vi "Controller Acquisition and Actuation Loop.vi"(4 "Iteration Duration":i64, 5 "Missed iteration?":bool, 6 "Initial Corrector Kick Vector":dbl[](array[numeric]), 7 "Sync Objects":T3, 8 "error in (no error)":errorcluster, 9 "PS Variables":T1, 10 "BPM Variables":T2, 11 "FOFB Configuration":T7={"FOFB Parameters"={"Network"={"FOFB Controller IP"="", "LNLS Control Network IP"="", "LNLS Control Network Power Supplies TCP Port"=0, "LNLS Control Network FOFB Configuration TCP Port"=0, "Data Server TCP Port"=0, "Monitoring Data TCP Port"=0, "Configuration GUI TCP Port"=0, "TCP Listening Timeout"=0}, "Fast Acquisition"={"Acquisition Period"=0, "Data Buffer Size"=0, "Monitoring Period"=0}, "Response Matrix Measurement"={"Step Amplitude"=0.0, "Time Between Steps"=0, "Step Duration"=0, "Number of Averages"=0}, "Correction Algorithm"={"Correction Period"=0, "Reference Orbit Path"=path "", "Response Matrix Path"=path "", "Correction Matrix Path"=path "", "Horizontal Correction Factor"=0.0, "Vertical Correction Factor"=0.0, "Beam Current FOFB Threshold"=0.0, "Decouple H-V"=FALSE, "Use Additional BPM LPF"=FALSE, "BPM LPF Cutoff"=0.0}, "Acquisition Network"=[], "Actuation Network"=[]}, "Number of Acquisition Chassis"=0, "Number of Actuation Chassis"=0, "Number of BPM Readings"=0, "BPM Reading Names"=[], "Selected BPM Readings"=[0, 1, 2, 3, 4, 5, 6, 7, 8, 9, 10, 11, 12, 13, 14, 15, 16, 17, 18, 19, 20, 21, 22, 23, 24, 25, 26, 27, 28, 29, 30, 31, 32, 33, 34, 35, 36, 37, 38, 39, 40, 41, 42, 43, 44, 45, 46, 47, 48, 49], "Number of Correctors"=0, "Corrector Names"=[], "Selected Correctors"=[0, 1, 2, 3, 4, 5, 6, 7, 8, 9, 10, 11, 12, 13, 14, 15, 16, 17, 18, 19, 20, 21, 22, 23, 24, 25, 26, 27, 28, 29, 30, 31, 32, 33, 34, 35, 36, 37, 38, 39, 40, 41, 42, 43, 44, 45, 46, 47, 48, 49], "Reference Orbit"=[], "Response Matrix"=[], "Correction Matrix"=[], "Acquisition Chassis Names"=[], "Actuation Chassis Names"=[], "Acquisition Variables"=[], "Actuation Variables"=[], "PS Matrix Mapping"=[], "Inverse PS Matrix Mapping"=[], "Response Matrix Beam Energy (MeV)"=0.0, "PID Parameters"=[], "BPM Planes"=[], "Corrector Planes"=[], "RMM Step Factor"=[]}) -> (0 "error out":errorcluster)   [LabVIEW 2011, in "Controller VIs.lvlib"]
doc: "Continuously performs acquisition of all input variables (BPM readings, Power Supply readings, etc.) and forwards data to the <b>Decimated Acquisition Loop</b>. Depending on the <b>Actuation State</b> (global variable), performs actuations coming from one of the following sources (global variables):\n\n<b>Actuation State</b> = Only Reading\n (no actuation)\n\n<b>Actuation State</b> = Manual\n PS_Manual_Setpoints\n\n<b>Actuation State</b> = FOFB, Initializing FOFB, Stopping FOFB\n PS_FOFB_Setpoints\n\n<b>Actuation State</b> = Response Matrix Measurement\n PS_RMM_Setpoints"
uses:
  Controller VIs.lvlib
  Types Definitions/Type FOFB Configuration.ctl
  Types Definitions/Type FOFB Parameters.ctl
  Types Definitions/Type Network Configuration.ctl
  Types Definitions/Type FA Configuration.ctl
  Types Definitions/Type Response Matrix Measurement Configuration.ctl
  Types Definitions/Type Correction Algorithm Configuration.ctl
  Types Definitions/Type Acquisition Network Configuration.ctl
  Types Definitions/Type Actuation Network Configuration.ctl
  Types Definitions/Type PID Parameters.ctl
  Types Definitions/Type Synchronization Objects.ctl
  Types Definitions/Type Blocking Synchronization Objects.ctl
  Types Definitions/Type FA Request Parameters.ctl
  Types Definitions/Type BPM and PS select cluster.ctl
  Types Definitions/Type FA File Parameters.ctl
  Types Definitions/Type Monitoring Data.ctl
  Types Definitions/Type Diagnostics Data.ctl
  Types Definitions/Type CPU Loads Array.ctl
  Types Definitions/Type CPU Loads.ctl
  Types Definitions/Type Non-blocking Synchronization Objects.ctl
  Types Definitions/Type FOFB Variables.ctl
  Types Definitions/Type Actuation State.ctl
  Types Definitions/Type BPM Variables.ctl
  Types Definitions/Type PS Variables.ctl
  <vilib>/Analysis/3filter.llb/Filter Passband Type.ctl
  Type Definitions.lvlib
  <vilib>/Analysis/NI_AALBase.lvlib
  <vilib>/ptbypt/NI_PtbyPt.lvlib
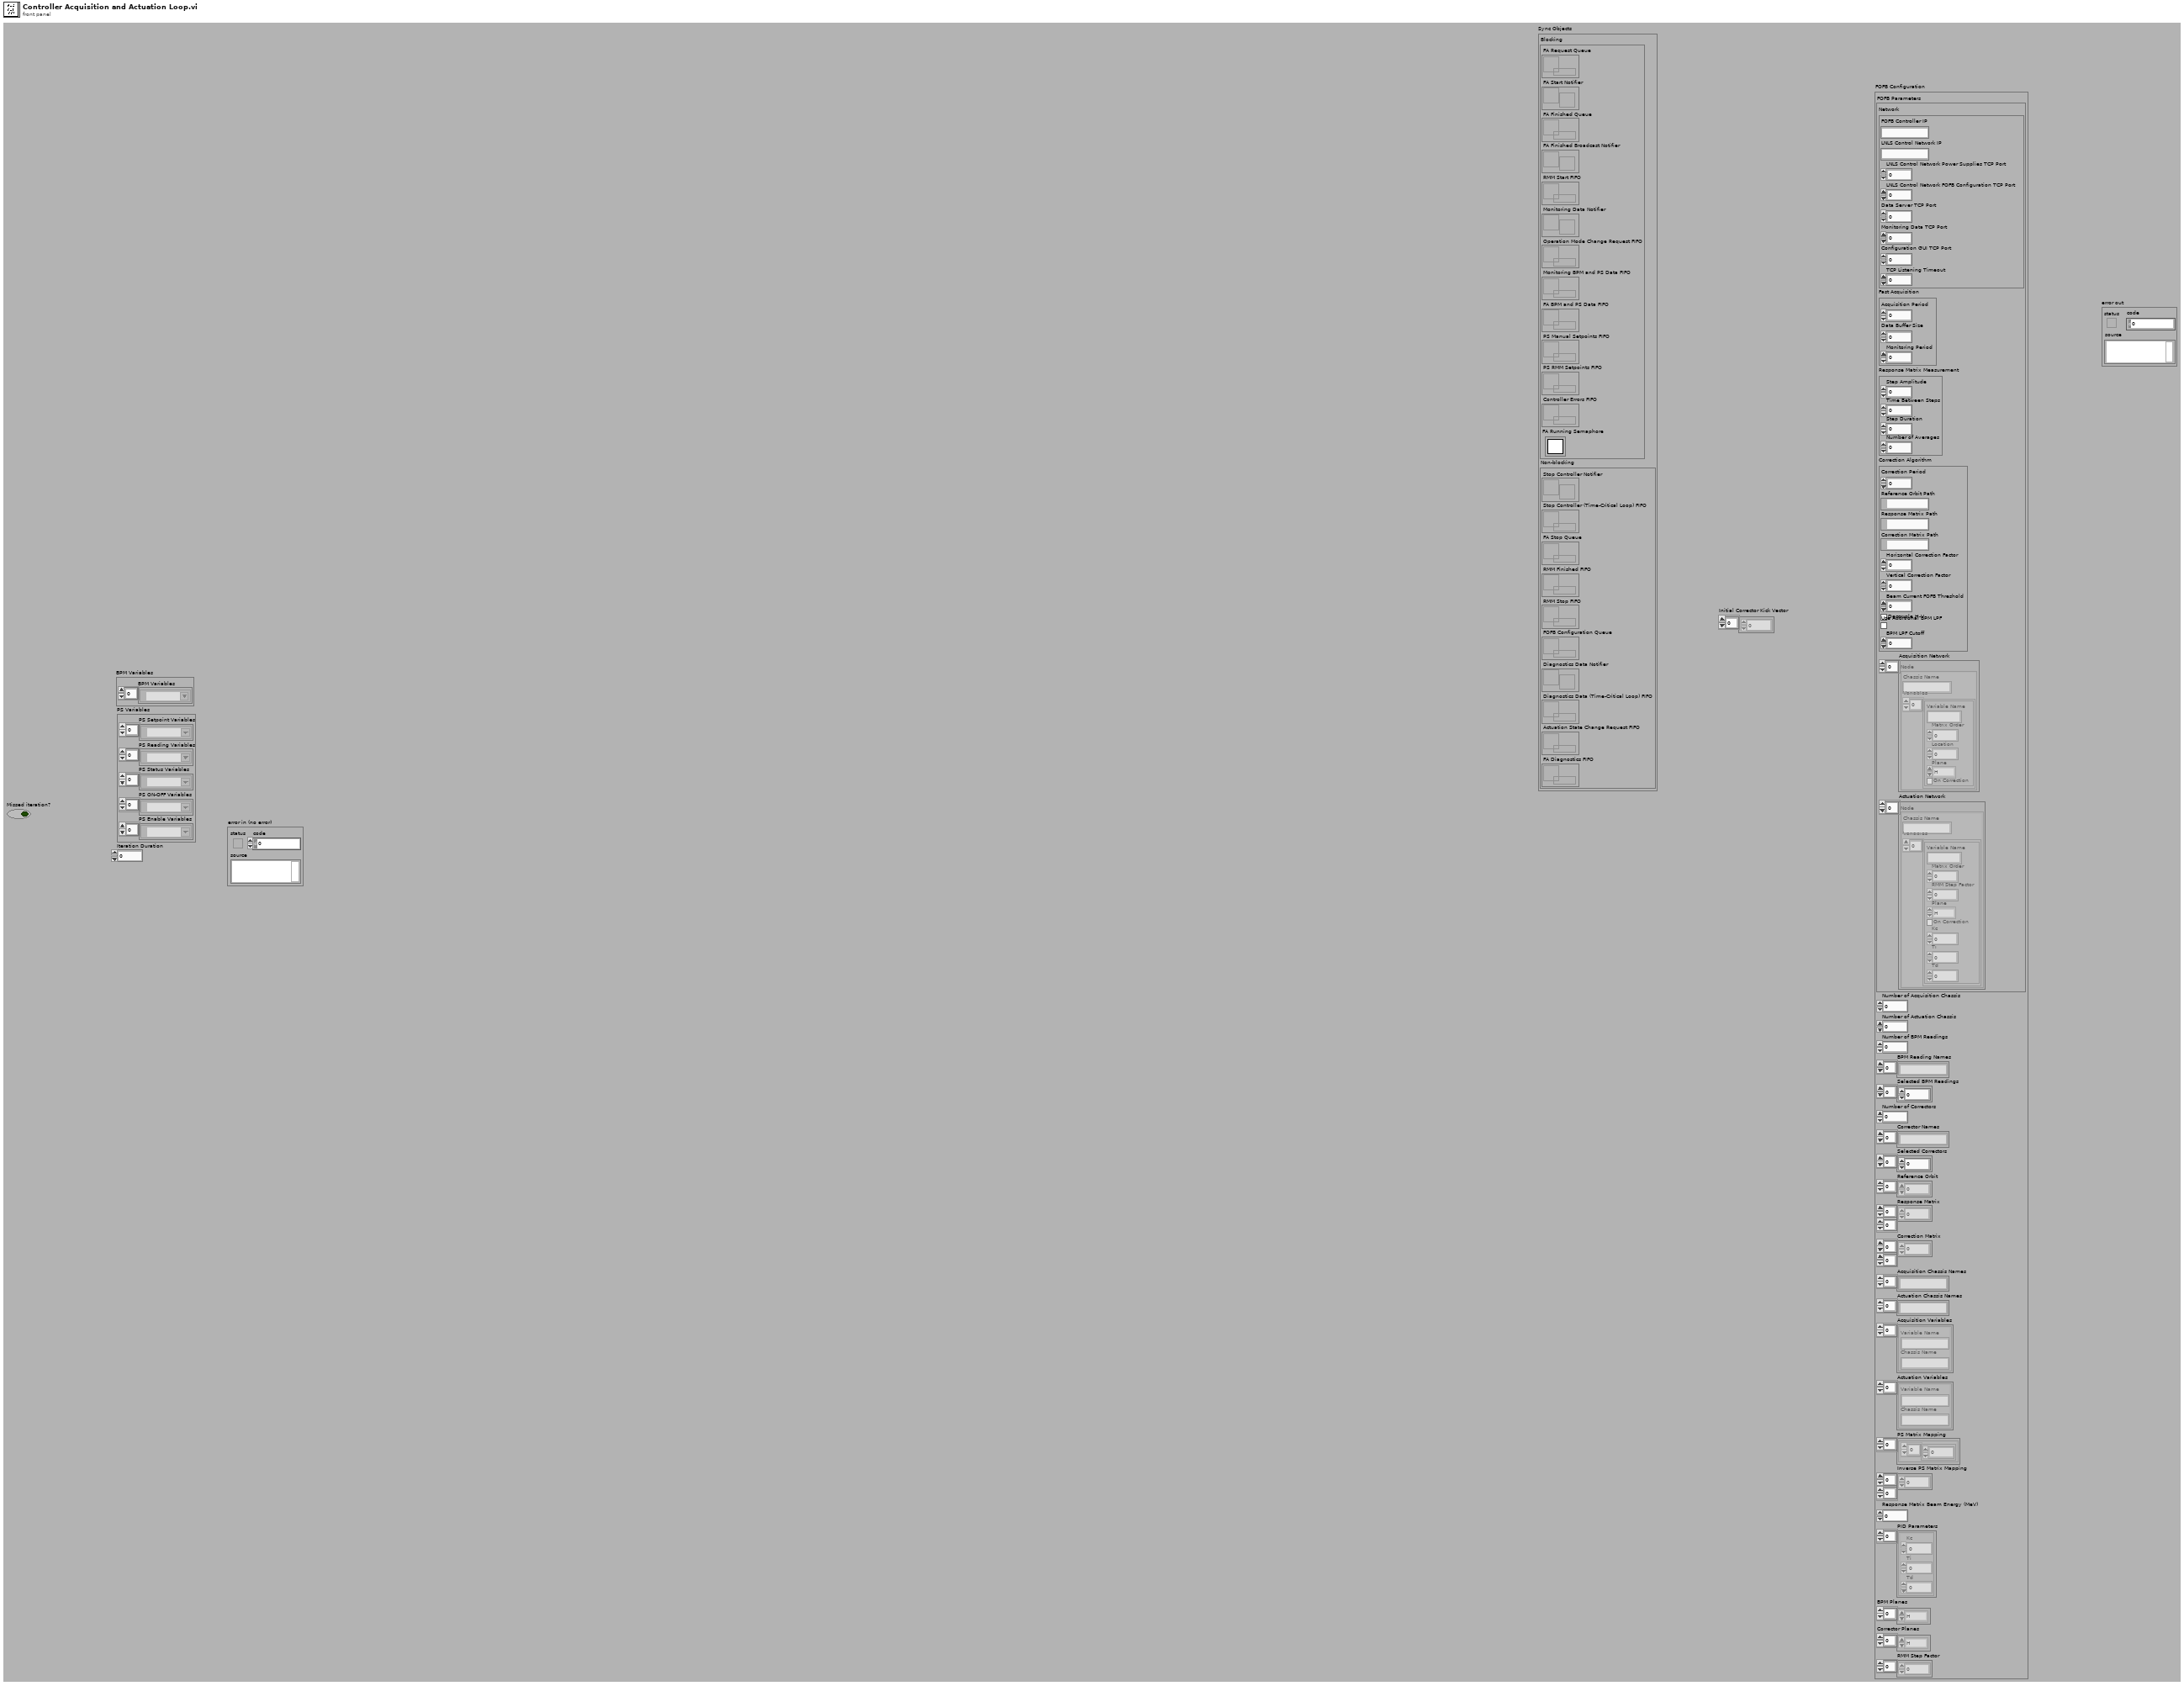
[diagram p1: front panel]
types:
  T1 = typedef "Type Definitions.lvlib/Type PS Variables.ctl" = cluster{"PS Setpoint Variables":refnum<k21>[], "PS Reading Variables":refnum<k21>[], "PS Status Variables":refnum<k21>[], "PS ON-OFF Variables":refnum<k21>[], "PS Enable Variables":refnum<k21>[]}
  T2 = typedef "Type Definitions.lvlib/Type BPM Variables.ctl" = cluster{"BPM Variables":refnum<k21>[]}
  T3 = typedef "Type Definitions.lvlib/Type Synchronization Objects.ctl" = cluster{"Blocking":T4, "Non-blocking":T6}
  T4 = typedef "Type Definitions.lvlib/Type Blocking Synchronization Objects.ctl" = cluster{"FA Request Queue":refnum<queue>, "FA Start Notifier":refnum<notifier>, "FA Finished Queue":refnum<queue>, "FA Finished Broadcast Notifier":refnum<notifier>, "RMM Start FIFO":refnum<k33>, "Monitoring Data Notifier":refnum<notifier>, "Operation Mode Change Request FIFO":refnum<k33>, "Monitoring BPM and PS Data FIFO":refnum<k33>, "FA BPM and PS Data FIFO":refnum<k33>, "PS Manual Setpoints FIFO":refnum<k33>, "PS RMM Setpoints FIFO":refnum<k33>, "Controller Errors FIFO":refnum<k33>, "FA Running Semaphore":T5}
  T5 = typedef "Semaphore RefNum" = refnum<k1>
  T6 = typedef "Type Definitions.lvlib/Type Non-blocking Synchronization Objects.ctl" = cluster{"Stop Controller Notifier":refnum<notifier>, "Stop Controller (Time-Critical Loop) FIFO":refnum<k33>, "FA Stop Queue":refnum<queue>, "RMM Finished FIFO":refnum<k33>, "RMM Stop FIFO":refnum<k33>, "FOFB Configuration Queue":refnum<queue>, "Diagnostics Data Notifier":refnum<notifier>, "Diagnostics Data (Time-Critical Loop) FIFO":refnum<k33>, "Actuation State Change Request FIFO":refnum<k33>, "FA Diagnostics FIFO":refnum<k33>}
  T7 = typedef "Type Definitions.lvlib/Type FOFB Configuration.ctl" = cluster{"FOFB Parameters":T8, "Number of Acquisition Chassis":i32, "Number of Actuation Chassis":i32, "Number of BPM Readings":i32, "BPM Reading Names":string[], "Selected BPM Readings":u32[], "Number of Correctors":i32, "Corrector Names":string[], "Selected Correctors":u32[], "Reference Orbit":dbl[], "Response Matrix":dbl[][], "Correction Matrix":dbl[][], "Acquisition Chassis Names":string[], "Actuation Chassis Names":string[], "Acquisition Variables":cluster{"Variable Name":string, "Chassis Name":string}[], "Actuation Variables":cluster{"Variable Name":string, "Chassis Name":string}[], "PS Matrix Mapping":cluster{u32[]}[], "Inverse PS Matrix Mapping":u32[][], "Response Matrix Beam Energy (MeV)":dbl, "PID Parameters":T15[], "BPM Planes":enum8{"H", "V"}[], "Corrector Planes":enum8{"H", "V"}[], "RMM Step Factor":dbl[]}
  T8 = typedef "Type Definitions.lvlib/Type FOFB Parameters.ctl" = cluster{"Network":T9, "Fast Acquisition":T10, "Response Matrix Measurement":T11, "Correction Algorithm":T12, "Acquisition Network":T13, "Actuation Network":T14}
  T9 = typedef "Type Definitions.lvlib/Type Network Configuration.ctl" = cluster{"FOFB Controller IP":string, "LNLS Control Network IP":string, "LNLS Control Network Power Supplies TCP Port":u16, "LNLS Control Network FOFB Configuration TCP Port":u16, "Data Server TCP Port":u16, "Monitoring Data TCP Port":u16, "Configuration GUI TCP Port":u16, "TCP Listening Timeout":i32}
  T10 = typedef "Type Definitions.lvlib/Type FA Configuration.ctl" = cluster{"Acquisition Period":u32, "Data Buffer Size":u32, "Monitoring Period":u32}
  T11 = typedef "Type Definitions.lvlib/Type Response Matrix Measurement Configuration.ctl" = cluster{"Step Amplitude":dbl, "Time Between Steps":u32, "Step Duration":u32, "Number of Averages":u32}
  T12 = typedef "Type Definitions.lvlib/Type Correction Algorithm Configuration.ctl" = cluster{"Correction Period":u32, "Reference Orbit Path":path, "Response Matrix Path":path, "Correction Matrix Path":path, "Horizontal Correction Factor":dbl, "Vertical Correction Factor":dbl, "Beam Current FOFB Threshold":dbl, "Decouple H-V":bool, "Use Additional BPM LPF":bool, "BPM LPF Cutoff":dbl}
  T13 = typedef "Type Definitions.lvlib/Type Acquisition Network Configuration.ctl" = cluster{"Chassis Name":string, "Variables":cluster{"Variable Name":string, "Matrix Order":u32, "Location":dbl, "Plane":enum8{"H", "V"}, "On Correction":bool}[]}[]
  T14 = typedef "Type Definitions.lvlib/Type Actuation Network Configuration.ctl" = cluster{"Chassis Name":string, "Variables":cluster{"Variable Name":string, "Matrix Order":u32, "RMM Step Factor":dbl, "Plane":enum8{"H", "V"}, "On Correction":bool, "Kc":dbl, "Ti":dbl, "Td":dbl}[]}[]
  T15 = typedef "Type Definitions.lvlib/Type PID Parameters.ctl" = cluster{"Kc":fxp<+/-,16,8>, "Ti":fxp<+/-,16,8>, "Td":fxp<+/-,16,8>}
  T16 = typedef "Type Definitions.lvlib/Type Actuation State.ctl" = enum16{"Only reading", "Manual", "FOFB Initialization", "FOFB", "FOFB Stopping", "RMM Initialization", "RMM", "RMM Stopping"}
  T17 = enum16{"Idle Mode", "Error Mode", "Manual Mode", "FOFB Mode", "RMM Mode"}
  T18 = typedef "NI_AALBase.lvlib/Filter Passband Type.ctl" = enum32{"Lowpass", "Highpass", "Bandpass", "Bandstop"}
  T19 = typedef "Type Definitions.lvlib/Type FOFB Variables.ctl" = cluster{"Correction Period":u32, "Reference Orbit":dbl[], "Response Matrix":dbl[][], "Correction Matrix":dbl[][], "Decouple H-V":bool, "Horizontal Correction Factor":dbl, "Vertical Correction Factor":dbl, "Selected BPM Readings":u32[], "Selected Correctors":u32[], "BPM Planes":enum8{"H", "V"}[], "Corrector Planes":enum8{"H", "V"}[], "Beam Current FOFB Threshold":dbl, "Response Matrix Beam Energy (MeV)":dbl}
  T20 = cluster{"filter structure":enum32{"IIR 2nd Order", "IIR 4th Order"}, "Reverse Coefficients":dbl[], "Forward Coefficients":dbl[]}
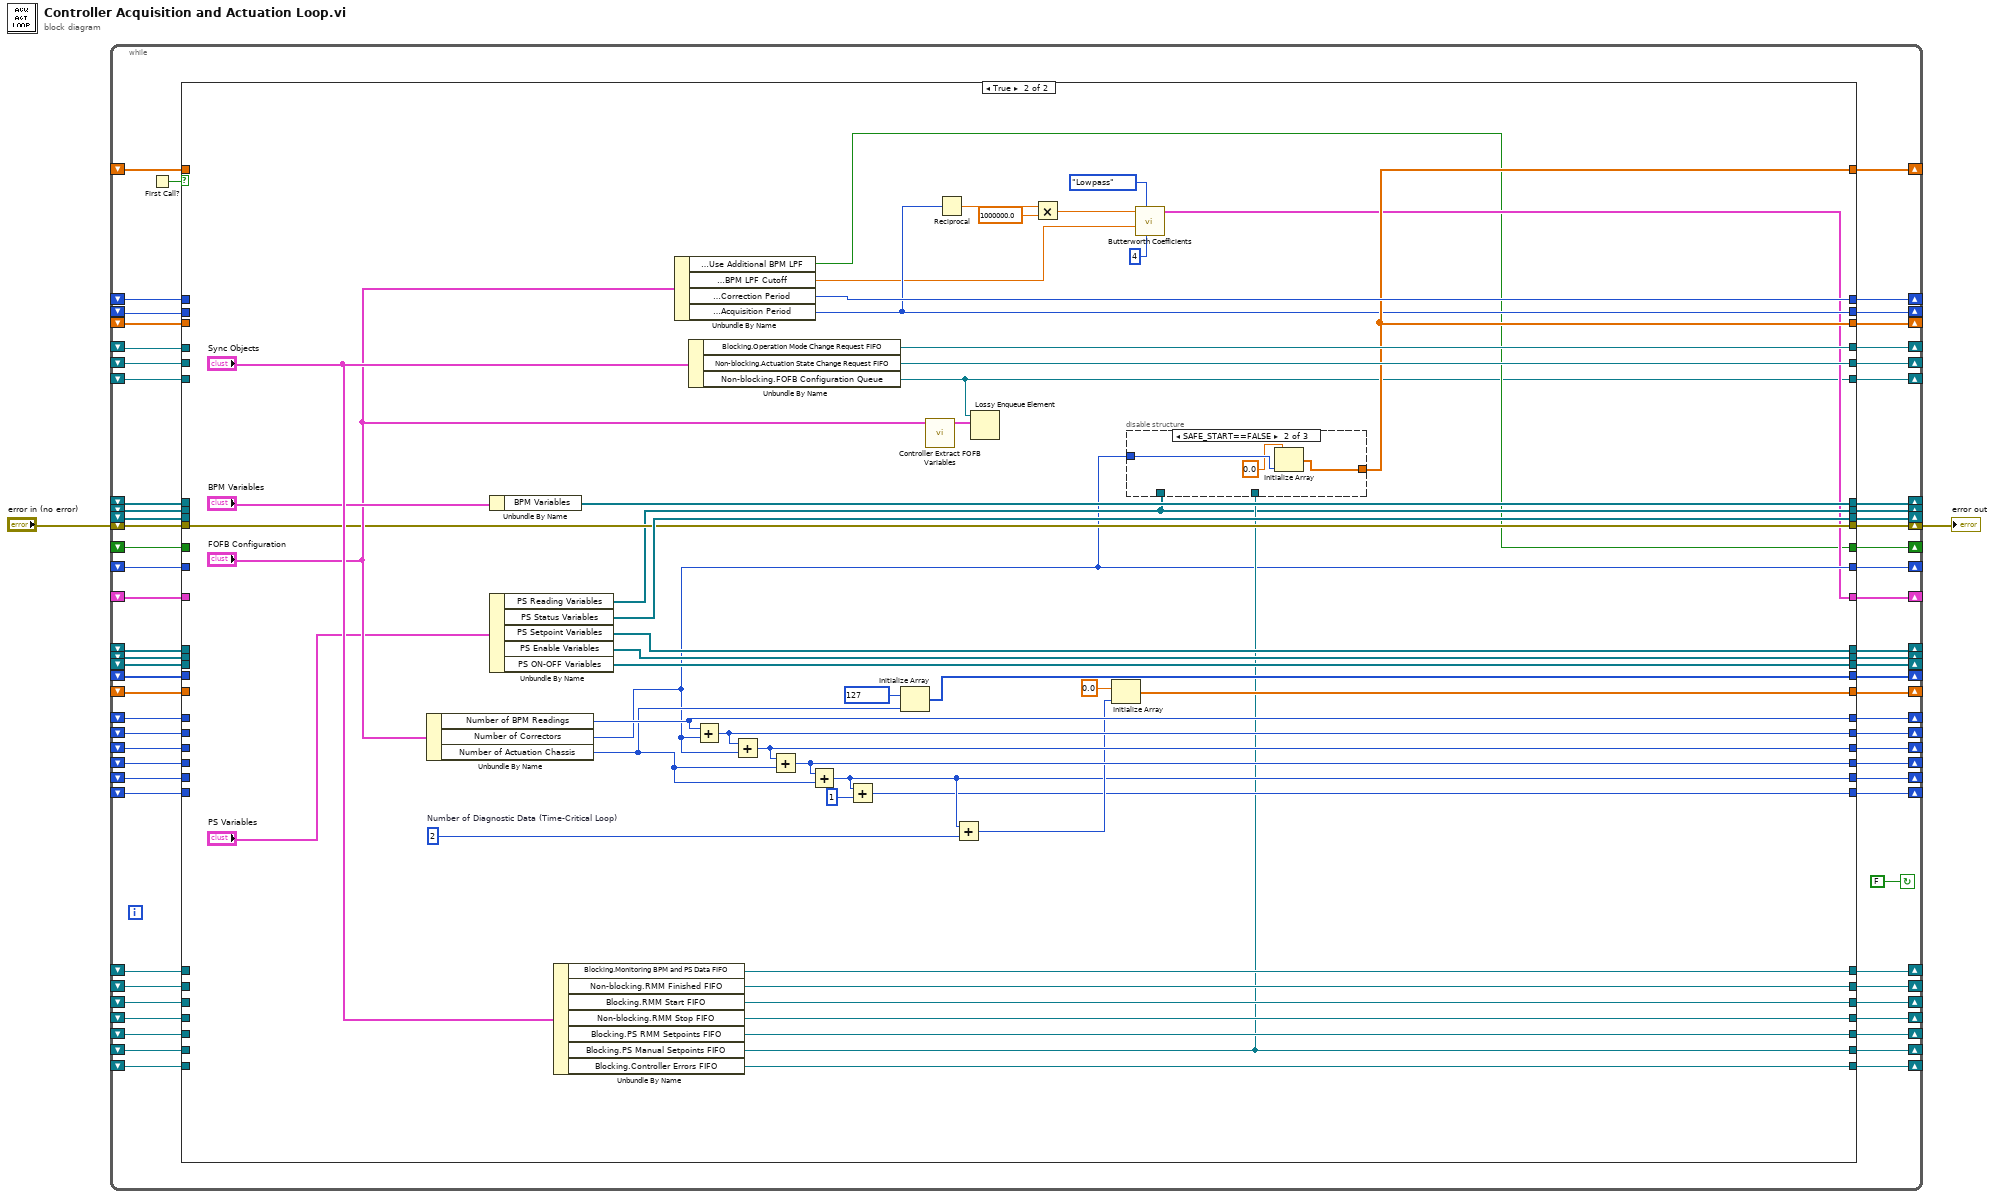
[diagram p0: block diagram]
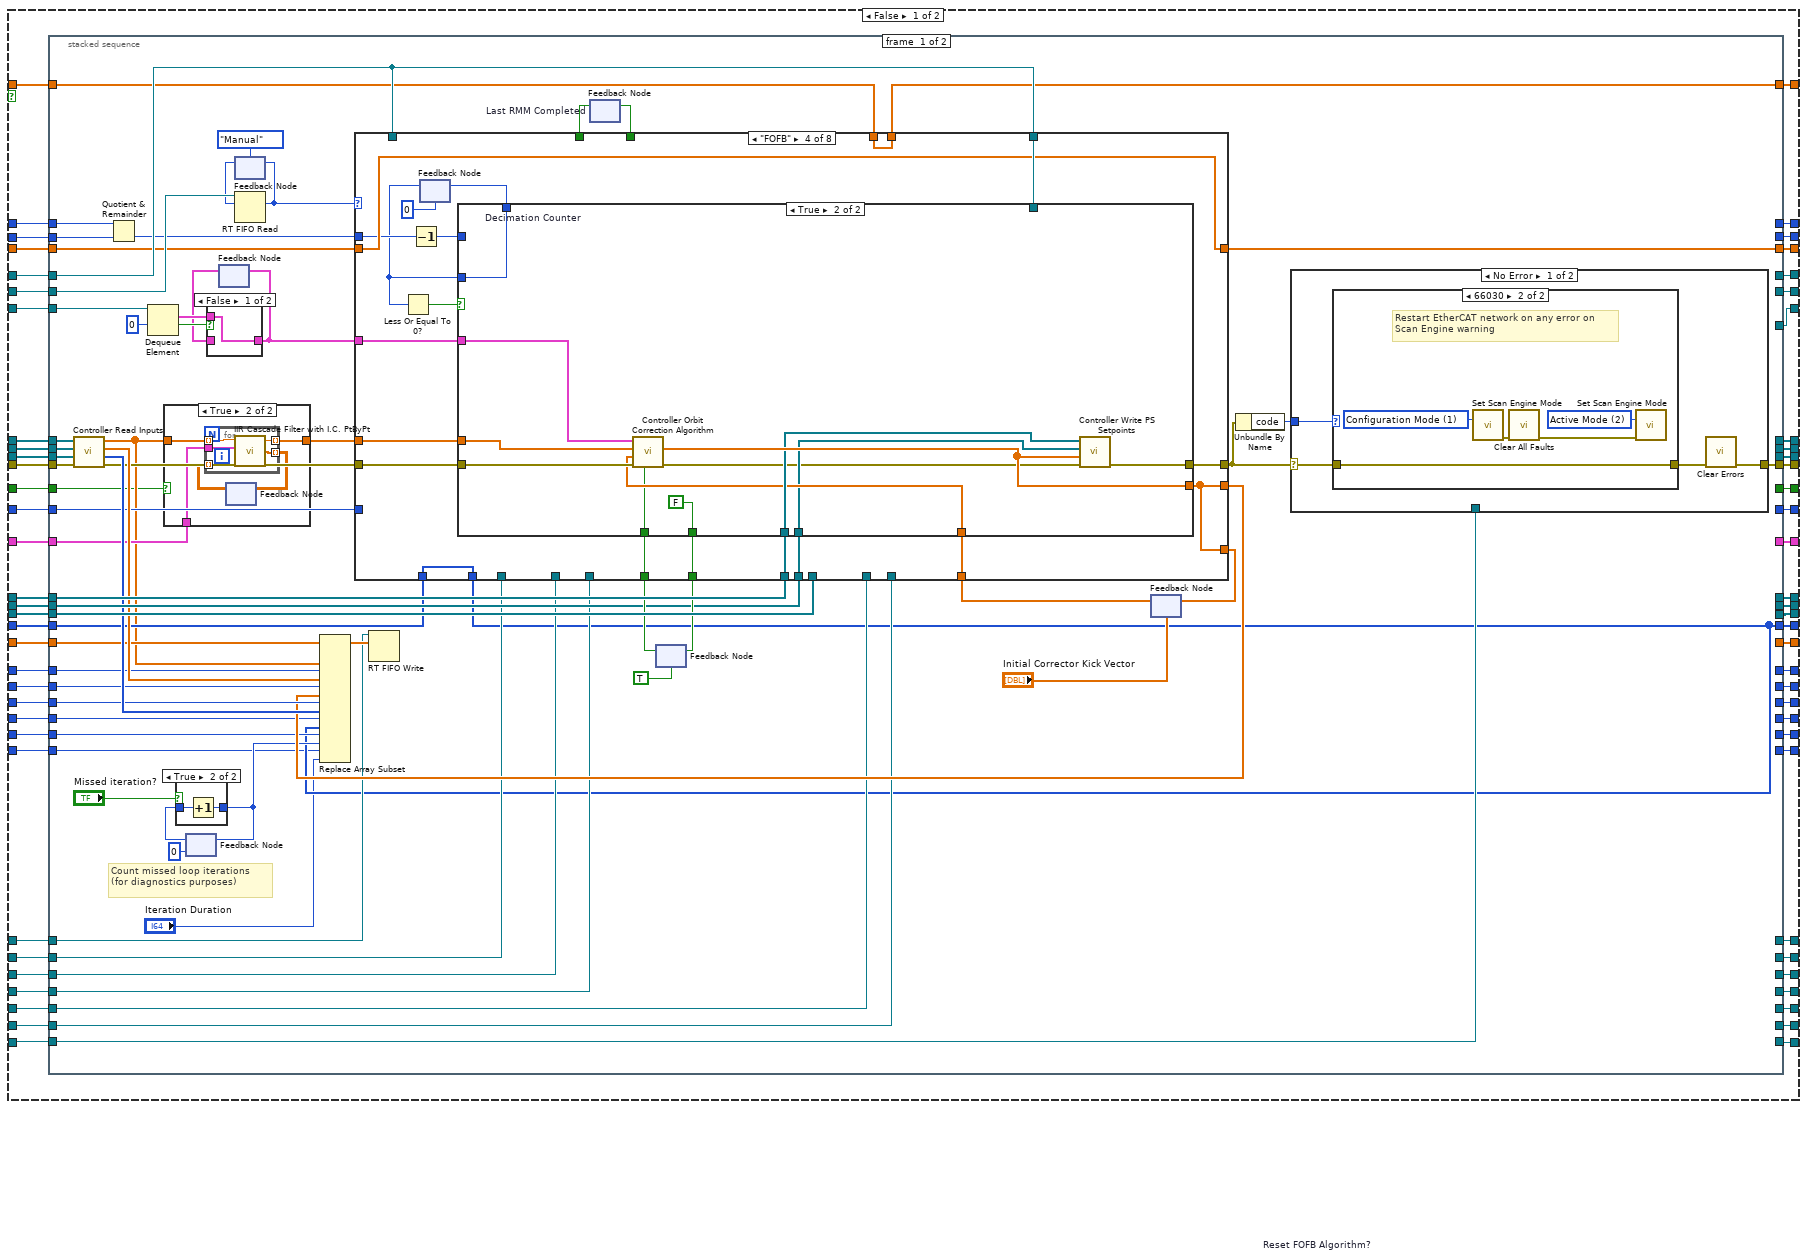
[diagram p2: hidden frame]
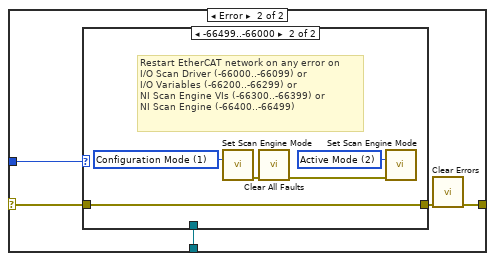
[diagram p6: hidden frame]
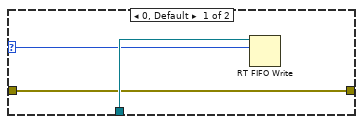
[diagram p7: hidden frame]
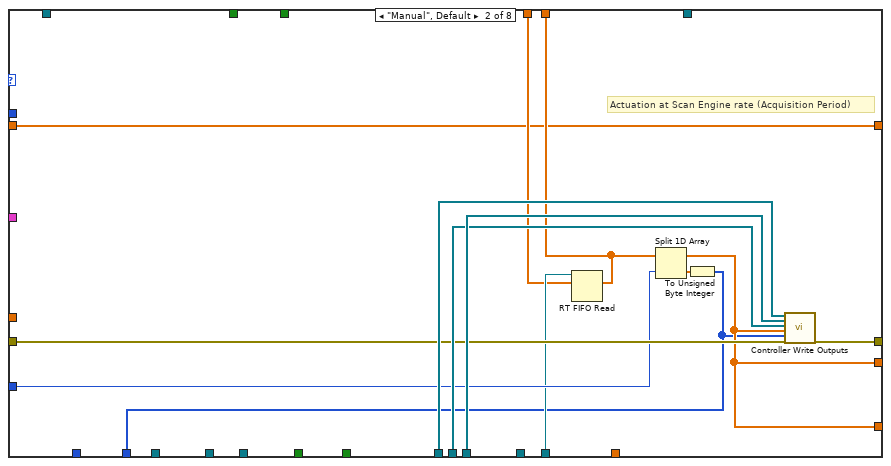
[diagram p9: hidden frame]
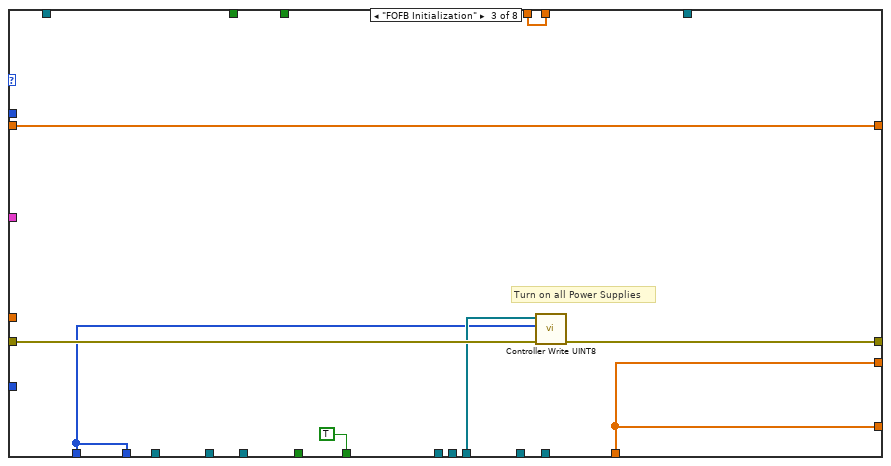
[diagram p10: hidden frame]
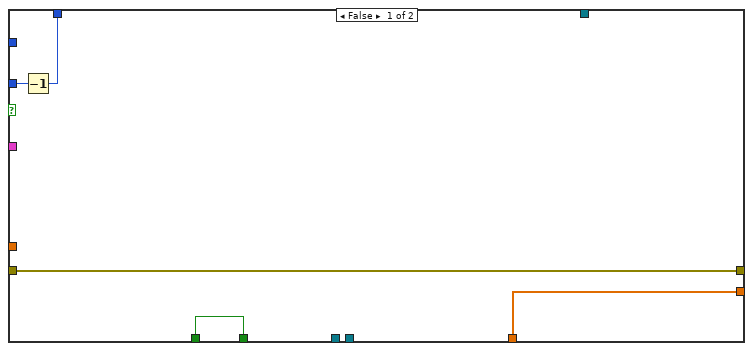
[diagram p11: hidden frame]
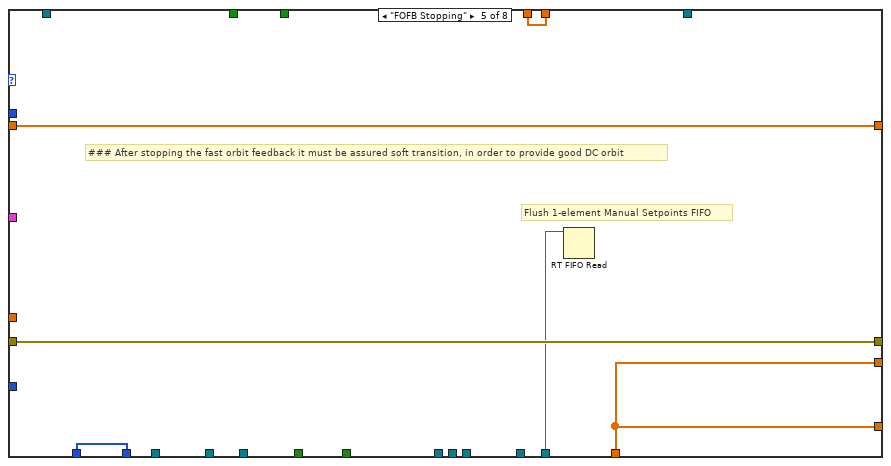
[diagram p12: hidden frame]
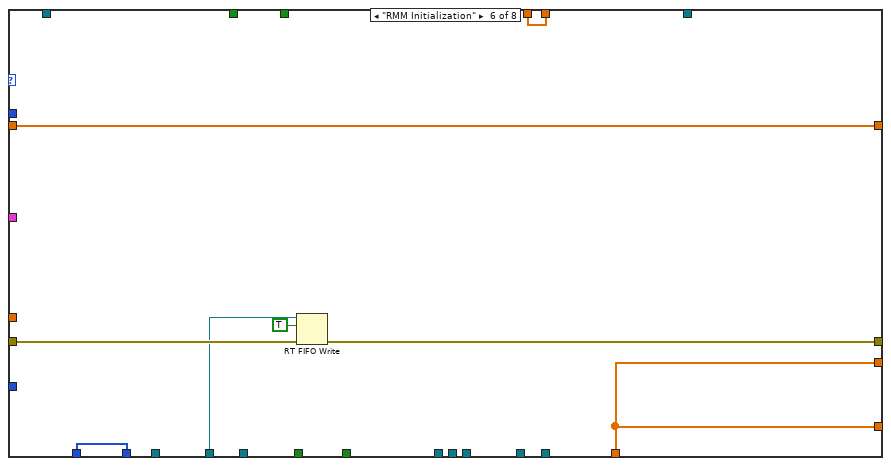
[diagram p13: hidden frame]
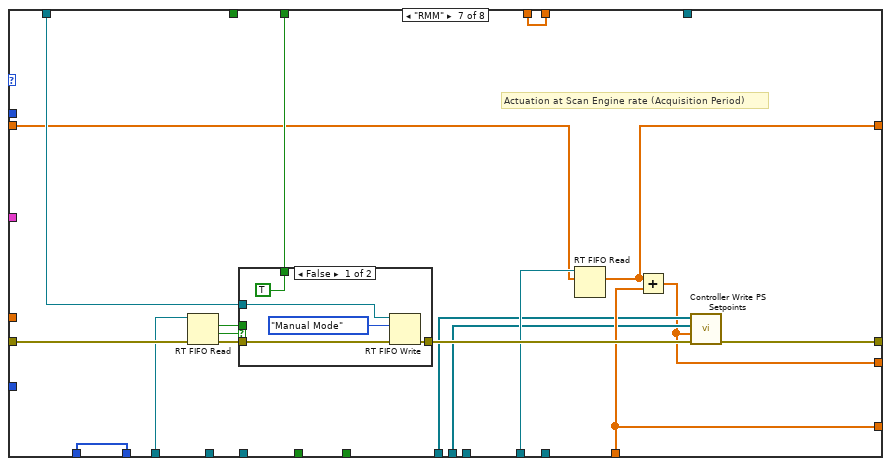
[diagram p14: hidden frame]
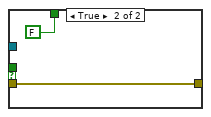
[diagram p15: hidden frame]
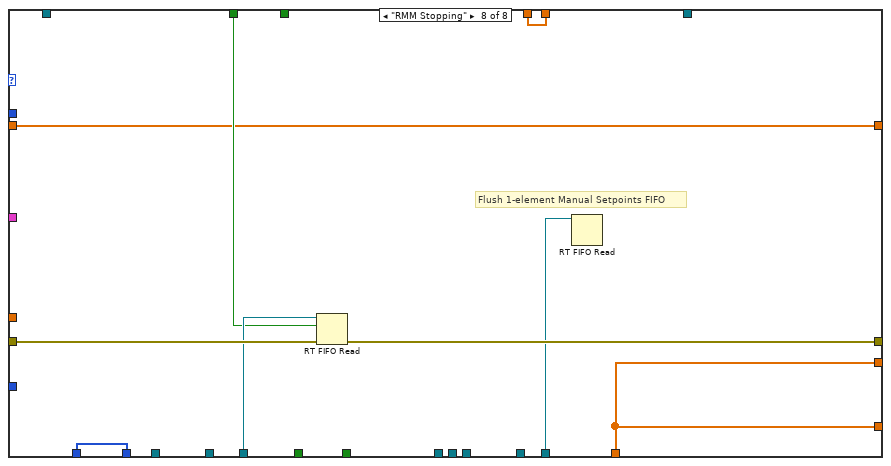
[diagram p16: hidden frame]
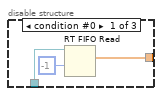
[diagram p19: hidden frame]
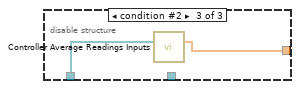
[diagram p20: hidden frame]
diagram:
  n1 = while {
    shift-right: [w52] -> w2
    shift-left: "error in (no error)" -> [w51]
    shift-right: [w47] -> _
    shift-left: _ -> [w59]
    shift-right: [w46] -> _
    shift-left: _ -> [w60]
    shift-right: [w45] -> _
    shift-left: _ -> [w62]
    shift-right: [w44] -> _
    shift-left: _ -> [w63]
    shift-right: [w43] -> _
    shift-left: _ -> [w68]
    shift-right: [w42] -> _
    shift-left: _ -> [w67]
    shift-right: [w41] -> _
    shift-left: _ -> [w65]
    shift-right: [w40] -> _
    shift-left: _ -> [w50]
    shift-right: [w39] -> _
    shift-left: _ -> [w64]
    shift-right: [w38] -> _
    shift-left: _ -> [w61]
    shift-right: [w37] -> _
    shift-left: _ -> [w66]
    shift-right: [w36] -> _
    shift-left: _ -> [w56]
    shift-right: [w35] -> _
    shift-left: _ -> [w58]
    shift-right: [w34] -> _
    shift-left: _ -> [w55]
    shift-right: [w33] -> _
    shift-left: _ -> [w57]
    shift-right: [w32] -> _
    shift-left: _ -> [w54]
    shift-right: [w31] -> _
    shift-left: _ -> [w53]
    shift-right: [w30] -> _
    shift-left: _ -> [w23]
    shift-right: [w29] -> _
    shift-left: _ -> [w22]
    shift-right: [w28] -> _
    shift-left: _ -> [w21]
    shift-right: [w27] -> _
    shift-left: _ -> [w20]
    shift-right: [w26] -> _
    shift-left: _ -> [w19]
    shift-right: [w25] -> _
    shift-left: _ -> [w18]
    shift-right: [w24] -> _
    shift-left: _ -> [w17]
    shift-right: [w15] -> _
    shift-left: _ -> [w16]
    shift-right: [w13] -> _
    shift-left: _ -> [w14]
    shift-right: [w11] -> _
    shift-left: _ -> [w12]
    shift-right: [w10] -> _
    shift-left: _ -> [w9]
    shift-right: [w8] -> _
    shift-left: _ -> [w7]
    shift-right: [w5] -> _
    shift-left: _ -> [w6]
    shift-right: [w4] -> _
    shift-left: _ -> [w3]
    stop <- FALSE continue-if-true
    n2 = First Call?() -> (First Call?: T/F=w48:bool)
    n3 = case shown="True" w48 {
      tunnel: w68 -> [w132 _]
      tunnel: w67 -> [w131 _]
      tunnel: w66 -> [w130 _]
      tunnel: w65 -> [w129 _]
      tunnel: w64 -> [w128 _]
      tunnel: w63 -> [w127 _]
      tunnel: w62 -> [w126 _]
      tunnel: w61 -> [w125 _]
      tunnel: w60 -> [w124 _]
      tunnel: w59 -> [w123 _]
      tunnel: w58 -> [w122 _]
      tunnel: w57 -> [w121 _]
      tunnel: w56 -> [w120 _]
      tunnel: w55 -> [w119 _]
      tunnel: w54 -> [w118 _]
      tunnel: w53 -> [w117 _]
      tunnel: [w116 w396] -> w52
      tunnel: w51 -> [w115 w396]
      tunnel: w50 -> [w114 _]
      tunnel: [w112 w425] -> w47
      tunnel: [w111 w389] -> w46
      tunnel: [w110 w424] -> w45
      tunnel: [w109 w423] -> w44
      tunnel: [w108 w422] -> w43
      tunnel: [w107 w390] -> w42
      tunnel: [w106 w421] -> w41
      tunnel: [w105 w387] -> w40
      tunnel: [w104 w420] -> w39
      tunnel: [w103 w419] -> w38
      tunnel: [w102 w418] -> w37
      tunnel: [w101 w417] -> w36
      tunnel: [w100 w416] -> w35
      tunnel: [w99 w415] -> w34
      tunnel: [w98 w414] -> w33
      tunnel: [w97 w413] -> w32
      tunnel: [w96 w395] -> w31
      tunnel: [w83 w403] -> w30
      tunnel: [w82 w402] -> w29
      tunnel: [w81 w401] -> w28
      tunnel: [w80 w400] -> w27
      tunnel: [w79 w399] -> w26
      tunnel: [w78 w391] -> w25
      tunnel: [w77 w398] -> w24
      tunnel: w23 -> [w89 _]
      tunnel: w22 -> [w88 _]
      tunnel: w21 -> [w87 _]
      tunnel: w20 -> [w84 _]
      tunnel: w19 -> [w85 _]
      tunnel: w18 -> [w86 _]
      tunnel: w17 -> [w113 _]
      tunnel: w16 -> [w95 _]
      tunnel: [w94 w397] -> w15
      tunnel: w14 -> [w93 _]
      tunnel: [w92 w392] -> w13
      tunnel: w12 -> [w91 _]
      tunnel: [w90 w392] -> w11
      tunnel: w9 -> [w76 _]
      tunnel: [w75 w393] -> w10
      tunnel: [w73 w378] -> w8
      tunnel: w7 -> [w74 _]
      tunnel: w6 -> [w72 _]
      tunnel: [w71 w383] -> w5
      tunnel: [w69 w380] -> w4
      tunnel: w3 -> [w70 _]
      frame False {
        n4 = stacked-sequence {
          tunnel: w132 -> [w199 w373]
          tunnel: w131 -> [w198 w372]
          tunnel: w130 -> [w197 w367]
          tunnel: w129 -> [w196 w371]
          tunnel: w128 -> [w192 w369]
          tunnel: w127 -> [w191 w374]
          tunnel: w126 -> [w190 w375]
          tunnel: w125 -> [w183 w368]
          tunnel: w124 -> [w182 w376]
          tunnel: w123 -> [w179 w377]
          tunnel: w122 -> [w176 w365]
          tunnel: w121 -> [w175 w363]
          tunnel: w120 -> [w174 w366]
          tunnel: w119 -> [w169 w364]
          tunnel: w118 -> [w168 w362]
          tunnel: w117 -> [w166 w361]
          tunnel: [w164 _] -> w116
          tunnel: w115 -> [w161 _]
          tunnel: w114 -> [w158 w370]
          tunnel: w87 -> [w157 w358]
          tunnel: w88 -> [w156 w359]
          tunnel: w89 -> [w155 w360]
          tunnel: w113 -> [w154 w354]
          tunnel: w86 -> [w153 w355]
          tunnel: w85 -> [w152 w356]
          tunnel: w84 -> [w151 w357]
          tunnel: [_ w377] -> w112
          tunnel: [_ w376] -> w111
          tunnel: [_ w375] -> w110
          tunnel: [_ w374] -> w109
          tunnel: [_ w373] -> w108
          tunnel: [_ w372] -> w107
          tunnel: [_ w371] -> w106
          tunnel: [_ w370] -> w105
          tunnel: [_ w369] -> w104
          tunnel: [_ w368] -> w103
          tunnel: [_ w367] -> w102
          tunnel: [_ w366] -> w101
          tunnel: [_ w365] -> w100
          tunnel: [_ w364] -> w99
          tunnel: [_ w363] -> w98
          tunnel: [_ w362] -> w97
          tunnel: [_ w361] -> w96
          tunnel: [_ w360] -> w83
          tunnel: [_ w359] -> w82
          tunnel: [_ w358] -> w81
          tunnel: [_ w357] -> w80
          tunnel: [_ w356] -> w79
          tunnel: [_ w355] -> w78
          tunnel: [_ w354] -> w77
          tunnel: w95 -> [w150 _]
          tunnel: [w149 _] -> w94
          tunnel: w93 -> [w148 _]
          tunnel: [w147 _] -> w92
          tunnel: w91 -> [w146 _]
          tunnel: [w145 _] -> w90
          tunnel: w76 -> [w143 w353]
          tunnel: [_ w353] -> w75
          tunnel: w74 -> [w142 w352]
          tunnel: [_ w352] -> w73
          tunnel: w72 -> [w141 w351]
          tunnel: [_ w351] -> w71
          tunnel: w70 -> [w138 w350]
          tunnel: [_ w350] -> w69
          frame #0 {
            # "Count missed loop iterations\n(for diagnostics purposes)"
            n5 = call "Controller Read Inputs.vi"("error in (no error)"=w161, "PS Status Variables"=w196, "PS Reading Variables"=w198, "BPM Variables"=w199) -> ("error out"=w160:errorcluster, "PS Status (per PS Rack)"=w177:u8[], "PS Readings"=w178:dbl[], "BPM Readings"=w139:dbl[])  [unwired: 4 in]
            n6 = Quotient & Remainder(x=w179, y=w182) -> (floor(x/y)=w181:u32)  [unwired: 1 out]
            n7 = Dequeue Element(queue=w142, timeout in ms (-1)=0) -> (element=w136:T19, timed out?=w137:bool)  [unwired: 1 in, 2 out]
            n8 = case shown="True" w138 {
              tunnel: w141 -> [_ w205]
              tunnel: [w202 w204] -> w140
              tunnel: w139 -> [w202 w203]
              frame False {
              }
              frame True {
                n9 = feedback #1() -> (w206:dbl[][])  [unwired: 1 in]
                n10 = for {
                  tunnel: [w212] -> w204 mode=indexing
                  tunnel: w206 -> [w211] mode=indexing
                  tunnel: [w210] -> w207 mode=indexing
                  tunnel: w205 -> [w209]
                  tunnel: w203 -> [w208] mode=indexing
                  n11 = call <vilib>:"IIR Cascade Filter with I.C. PtByPt.vi"("x"=w208, "IIR Filter Cluster"=w209, "Initial Condition"=w211) -> ("Filtered x"=w212:dbl, "Final Condition"=w210:dbl[])  [unwired: 2 in, 1 out]
                }
                n12 = feedback-in #1(w207) -> ()
              }
            }
            n13 = feedback #2(u32 0) -> (w194:u32)
            n14 = case shown="True" "Missed iteration?" {
              tunnel: [w347 w349] -> w167
              tunnel: w194 -> [w347 w348]
              frame False {
              }
              frame True {
                n15 = Increment(x=w348) -> (x+1=w349:u32)
              }
            }
            n16 = feedback-in #2(w167) -> ()
            n17 = feedback #3() -> (w134:T19)  [unwired: 1 in]
            n18 = case shown="False" w137 {
              tunnel: [w200 w201] -> w133
              tunnel: w136 -> [w200 _]
              tunnel: w134 -> [_ w201]
              frame False {
              }
              frame True {
              }
            }
            n19 = feedback-in #3(w133) -> ()
            n20 = feedback #4(Type_Actuation_State."Manual" ("Actuation State")) -> (w163:T16)
            n21 = RT FIFO Read(0:w191, 1:w163) -> (9:w180:T16)  [unwired: 2 in, 4 out]
            n22 = feedback-in #4(w180) -> ()
            n23 = feedback #5 "Last RMM Completed"() -> (w188:bool)  [unwired: 1 in]
            n24 = feedback #6 "Reset FOFB Algorithm?"(TRUE ("x")) -> (w185:bool)
            n25 = feedback #7("Initial Corrector Kick Vector") -> (w193:dbl[])
            n26 = case shown="\"FOFB\"" w180 {
              tunnel: [w240 w250 w258 w281 w304 w310 w330 w345] -> w159
              tunnel: w160 -> [w240 w249 w259 w280 w304 w312 w329 w346]
              tunnel: w140 -> [_ _ _ w279 _ _ _ _]
              tunnel: w192 -> [_ w253 _ w278 _ _ w318 _]
              tunnel: w197 -> [_ w252 w257 _ _ _ _ _]
              tunnel: w181 -> [_ _ _ w264 _ _ _ _]
              tunnel: [w239 w248 w260 w271 w303 w309 w324 w342] -> w187
              tunnel: w193 -> [w239 _ w260 w277 w303 w309 w324 w342]
              tunnel: w190 -> [_ _ _ w276 _ _ _ _]
              tunnel: w157 -> [_ _ _ _ _ w311 _ _]
              tunnel: w156 -> [_ _ _ _ _ _ w328 _]
              tunnel: w190 -> [_ _ _ _ _ _ w327 _]
              tunnel: w151 -> [_ _ _ _ _ _ _ w344]
              tunnel: [_ _ _ _ _ _ w323 _] -> w189
              tunnel: w188 -> [_ _ _ _ _ _ _ w343]
              tunnel: w185 -> [_ _ _ w275 _ _ _ _]
              tunnel: [_ _ TRUE ("Good value?") w273 _ _ _ _] -> w184
              tunnel: w183 -> [_ w251 _ w274 _ _ w317 _]
              tunnel: [w239 w248 w260 w271 w303 w309 w316 w342] -> w170
              tunnel: w152 -> [_ _ _ _ _ _ w320 _]
              tunnel: w158 -> [_ w246 _ _ _ _ _ _]
              tunnel: w153 -> [_ w245 _ _ w299 _ _ w338]
              tunnel: [w238 w244 w254 w270 w302 w307 w319 w341] -> w149
              tunnel: w150 -> [w238 _ w254 w270 w302 w307 w319 w341]
              tunnel: w133 -> [_ _ _ w268 _ _ _ _]
              tunnel: [w237 w243 w256 w267 w301 w306 w315 w340] -> w147
              tunnel: w148 -> [w237 w242 w256 w267 w301 w306 w315 w340]
              tunnel: w146 -> [w236 w241 w255 w266 w300 w305 w314 w339]
              tunnel: [w236 w241 w255 w266 w300 w305 w313 w339] -> w145
              frame "Only reading" {
              }
              frame "Manual", Default {
                # "Actuation at Scan Engine rate (Acquisition Period)"
                n27 = RT FIFO Read(0:w245, 1:w242) -> (9:w243:dbl[])  [unwired: 2 in, 4 out]
                n28 = Split 1D Array(array=w243, index=w246) -> (first subarray=w248:dbl[], second subarray=w247:dbl[])
                n29 = To Unsigned Byte Integer(number=w247) -> (unsigned 8bit integer=w244:u8[])
                n30 = call "Controller Write Outputs.vi"("PS Setpoint Variables"=w253, "PS ON-OFF Variables"=w252, "PS Enable Variables"=w251, "PS Setpoints"=w248, "PS ON-OFF (per PS Rack)"=w244, "error in (no error)"=w249) -> ("error out"=w250:errorcluster)  [unwired: 13 in]
              }
              frame "FOFB Initialization" {
                # "Turn on all Power Supplies"
                n31 = call "Controller Write UINT8.vi"("error in (no error)"=w259, "Values"=w254, "Variables"=w257) -> ("error out"=w258:errorcluster)  [unwired: 8 in]
              }
              frame "FOFB" {
                n32 = Decrement(x=w264) -> (x-1=w272:u32)
                n33 = feedback #8 "Decimation Counter"(u32 0) -> (w263:u32)
                n34 = Less Or Equal To 0?(x=w263) -> (x <= 0?=w262:bool)
                n35 = case shown="True" w262 {
                  tunnel: [w286 w298] -> w281
                  tunnel: w280 -> [w286 w297]
                  tunnel: w279 -> [_ w290]
                  tunnel: w263 -> [w283 w287]
                  tunnel: w272 -> [_ _]
                  tunnel: w278 -> [_ w295]
                  tunnel: [w285 w296] -> w271
                  tunnel: w277 -> [w285 w294]
                  tunnel: w276 -> [_ _]
                  tunnel: w275 -> [w284 w289]
                  tunnel: w274 -> [_ w293]
                  tunnel: [w284 FALSE ("x")] -> w273
                  tunnel: [w282 w287] -> w269
                  tunnel: w268 -> [_ w288]
                  frame False {
                    n36 = Decrement(x=w283) -> (x-1=w282:u32)
                  }
                  frame True {
                    n37 = call "Controller Orbit Correction Algorithm.vi"("Resest?"=w289, "error in (no error)"=w297, "Initial Corrector Kick Vector"=w294, "Beam Position Vector"=w290, "FOFB Variables"=w288) -> ("error out"=w292:errorcluster, "Corrector Kick Vector"=w296:dbl[])  [unwired: 4 in, 1 out]
                    n38 = call "Controller Write PS Setpoints.vi"("PS Setpoint Variables"=w295, "PS Enable Variables"=w293, "PS Setpoints"=w296, "error in (no error)"=w292) -> ("error out"=w298:errorcluster)  [unwired: 6 in]
                  }
                }
                n39 = feedback-in #8(w269) -> ()
              }
              frame "FOFB Stopping" {
                # "Flush 1-element Manual Setpoints FIFO"
                # "### After stopping the fast orbit feedback it must be assured soft transition, in order to provide good DC orbit"
                n40 = RT FIFO Read(0:w299) -> ()  [unwired: 3 in, 5 out]
              }
              frame "RMM Initialization" {
                n41 = RT FIFO Write(0:w311, 1:TRUE ("notification"), 3:w312) -> (11:w310:errorcluster)  [unwired: 2 in, 3 out]
              }
              frame "RMM" {
                # "Actuation at Scan Engine rate (Acquisition Period)"
                n42 = RT FIFO Read(0:w328, 3:w329) -> (9:w322:bool, 10:w321:bool, 11:w326:errorcluster)  [unwired: 2 in, 2 out]
                n43 = case shown="False" w321 {
                  tunnel: w327 -> [w335 _]
                  tunnel: w326 -> [w334 w337]
                  tunnel: [w333 w337] -> w325
                  tunnel: [TRUE ("x") FALSE ("x")] -> w323
                  tunnel: w322 -> [_ _]
                  frame False {
                    n44 = RT FIFO Write(0:w335, 1:T17."Manual Mode" ("element"), 3:w334) -> (11:w333:errorcluster)  [unwired: 2 in, 3 out]
                  }
                  frame True {
                  }
                }
                n45 = RT FIFO Read(0:w320, 1:w314) -> (9:w313:dbl[])  [unwired: 2 in, 4 out]
                n46 = Add(x=w313, y=w324) -> (x+y=w316:dbl[])
                n47 = call "Controller Write PS Setpoints.vi"("PS Setpoint Variables"=w318, "PS Enable Variables"=w317, "PS Setpoints"=w316, "error in (no error)"=w325) -> ("error out"=w330:errorcluster)  [unwired: 6 in]
              }
              frame "RMM Stopping" {
                # "Flush 1-element Manual Setpoints FIFO"
                n48 = RT FIFO Read(0:w344, 1:w343, 3:w346) -> (11:w345:errorcluster)  [unwired: 1 in, 4 out]
                n49 = RT FIFO Read(0:w338) -> ()  [unwired: 3 in, 5 out]
              }
            }
            n50 = Replace Array Subset(array=w174, new element #1=w139, new element #2=w178, index #2=w176, new element #3=w170, index #3=w169, new element #4=w177, index #4=w175, new element #5=w149, index #5=w168, new element #6=w167, index #6=w166, new element #7="Iteration Duration", index #7=w143) -> (w172:dbl[])  [unwired: 1 in]
            n51 = RT FIFO Write(0:w155, 1:w172) -> ()  [unwired: 3 in, 4 out]
            n52 = feedback-in #5(w189) -> ()
            n53 = feedback-in #6(w184) -> ()
            n54 = feedback-in #7(w187) -> ()
            n55 = Unbundle By Name(w159) -> ("code"=w173:i32)
            n56 = case shown="No Error" w159 {
              selector: w159 -> [w216 w225]
              tunnel: w154 -> [_ w227]
              tunnel: w173 -> [w215 w226]
              tunnel: [w213 w223] -> w164
              frame No Error {
                n57 = case shown="66030" w215 {
                  tunnel: [w217 w218] -> w214
                  tunnel: w216 -> [w217 w218]
                  frame 0, Default {
                  }
                  frame 66030 {
                    w220 = 2 items=["Configuration Mode"=1, "Active Mode"=2] ("mode (Active Mode)")
                    w221 = 1 items=["Configuration Mode"=1, "Active Mode"=2] ("mode (Active Mode)")
                    # "Restart EtherCAT network on any error on \nScan Engine warning"
                    n58 = call <vilib>:"Set Scan Engine Mode.vi"("mode (Active Mode)"=w221) -> ("error out"=w222:errorcluster)  [unwired: 14 in]
                    n59 = call <vilib>:"Clear All Faults.vi"("error in (no error)"=w222) -> ("error out"=w219:errorcluster)  [unwired: 1 in, 9 out]
                    n60 = call <vilib>:"Set Scan Engine Mode.vi"("mode (Active Mode)"=w220, "error in (no error)"=w219) -> ()  [unwired: 13 in, 1 out]
                  }
                }
                n61 = call <vilib>:"Clear Errors.vi"("error in (no error)"=w214) -> ("error out"=w213:errorcluster)  [unwired: 6 in]
              }
              frame Error {
                n62 = case shown="-66499..-66000" w226 {
                  selector: w226 -> [w229 _]
                  tunnel: [w228 w231] -> w224
                  tunnel: w227 -> [w230 _]
                  tunnel: w225 -> [w228 w231]
                  frame 0, Default {
                    n63 = RT FIFO Write(0:w230, 1:w229) -> ()  [unwired: 3 in, 4 out]
                  }
                  frame -66499..-66000 {
                    w233 = 2 items=["Configuration Mode"=1, "Active Mode"=2] ("mode (Active Mode)")
                    w234 = 1 items=["Configuration Mode"=1, "Active Mode"=2] ("mode (Active Mode)")
                    # "Restart EtherCAT network on any error on \nI/O Scan Driver\t(-66000..-66099) or\nI/O Variables\t(-66200..-66299) or\nNI Scan Engine VIs\t(-66300..-66399) or\nNI Scan Engine (-66400..-66499)"
                    n64 = call <vilib>:"Set Scan Engine Mode.vi"("mode (Active Mode)"=w234) -> ("error out"=w235:errorcluster)  [unwired: 14 in]
                    n65 = call <vilib>:"Clear All Faults.vi"("error in (no error)"=w235) -> ("error out"=w232:errorcluster)  [unwired: 1 in, 9 out]
                    n66 = call <vilib>:"Set Scan Engine Mode.vi"("mode (Active Mode)"=w233, "error in (no error)"=w232) -> ()  [unwired: 13 in, 1 out]
                  }
                }
                n67 = call <vilib>:"Clear Errors.vi"("error in (no error)"=w224) -> ("error out"=w223:errorcluster)  [unwired: 6 in]
              }
            }
          }
          frame #1 {
          }
        }
      }
      frame True {
        w411 = 2  # Number of Diagnostic Data (Time-Critical Loop)
        n68 = Unbundle By Name("FOFB Configuration") -> ("Number of BPM Readings"=w416:i32, "Number of Correctors"=w387:i32, "Number of Actuation Chassis"=w408:i32)
        n69 = Unbundle By Name("BPM Variables") -> ("BPM Variables"=w422:refnum<k21>[])
        n70 = Unbundle By Name("PS Variables") -> ("PS Reading Variables"=w390:refnum<k21>[], "PS Status Variables"=w421:refnum<k21>[], "PS Setpoint Variables"=w420:refnum<k21>[], "PS Enable Variables"=w419:refnum<k21>[], "PS ON-OFF Variables"=w418:refnum<k21>[])
        n71 = Unbundle By Name("Sync Objects") -> ("Blocking.Monitoring BPM and PS Data FIFO"=w403:refnum<k33>, "Non-blocking.RMM Finished FIFO"=w402:refnum<k33>, "Blocking.RMM Start FIFO"=w401:refnum<k33>, "Non-blocking.RMM Stop FIFO"=w400:refnum<k33>, "Blocking.PS RMM Setpoints FIFO"=w399:refnum<k33>, "Blocking.PS Manual Setpoints FIFO"=w391:refnum<k33>, "Blocking.Controller Errors FIFO"=w398:refnum<k33>)
        n72 = Unbundle By Name("FOFB Configuration") -> ("FOFB Parameters.Correction Algorithm.Use Additional BPM LPF"=w380:bool, "FOFB Parameters.Correction Algorithm.BPM LPF Cutoff"=w381:dbl, "FOFB Parameters.Correction Algorithm.Correction Period"=w425:u32, "FOFB Parameters.Fast Acquisition.Acquisition Period"=w389:u32)
        n73 = Unbundle By Name("Sync Objects") -> ("Blocking.Operation Mode Change Request FIFO"=w424:refnum<k33>, "Non-blocking.Actuation State Change Request FIFO"=w423:refnum<k33>, "Non-blocking.FOFB Configuration Queue"=w378:refnum<queue>)
        n74 = Add(x=w416, y=w387) -> (x+y=w415:i32)
        n75 = Add(x=w415, y=w387) -> (x+y=w414:i32)
        n76 = Add(x=w414, y=w408) -> (x+y=w413:i32)
        n77 = Add(x=w413, y=w408) -> (x+y=w395:i32)
        n78 = Add(x=w395, y=1) -> (x+y=w393:i32)
        n79 = Initialize Array(u8 127, w408) -> (w397:u8[])
        n80 = call "Controller Extract FOFB Variables.vi"("FOFB Configuration"="FOFB Configuration") -> ("FOFB Variables"=w379:T19)  [unwired: 9 in, 1 out]
        n81 = Reciprocal(x=w389) -> (1/x=w385:dbl)
        n82 = Add(x=w395, y=w411) -> (x+y=w410:i32)
        n83 = Lossy Enqueue Element(queue=w378, element=w379) -> ()  [unwired: 1 in, 4 out]
        n84 = Multiply(x=w385, y=1000000.0) -> (x*y=w384:dbl)
        n85 = Initialize Array(0.0 ("element"), w410) -> (w417:dbl[])
        n86 = disable-structure shown="SAFE_START==FALSE" {
          disable-tunnel: [w428 w431 w433] -> w392
          disable-tunnel: w391 -> [w427 _ _]
          disable-tunnel: w387 -> [_ w430 _]
          disable-tunnel: w390 -> [_ _ w432]
          frame condition #0 {
            n87 = RT FIFO Read(0:w427, 2:-1 ("timeout in ms (0)")) -> (9:w428:dbl[])  [unwired: 2 in, 4 out]
          }
          frame condition #1 (active) {
            n88 = Initialize Array(0.0, w430) -> (w431:dbl[])
          }
          frame condition #2 {
            n89 = call "Controller Average Readings Inputs.vi"("PS Reading Variables"=w432) -> ("PS"=w433:dbl[])  [unwired: 11 in, 3 out]
          }
        }
        n90 = call <vilib>:"Butterworth Coefficients.vi"("order"=4, "filter type"=Filter_Passband_Type."Lowpass", "low cutoff freq: fl"=w381, "sampling freq: fs"=w384) -> ("IIR Filter Cluster"=w383:T20)  [unwired: 6 in, 1 out]
      }
    }
  }
  "error out" <- w2
